vi "move_backlash.vi"(6 "Axis enable":bool[](array[boolean])=[TRUE, TRUE, TRUE, TRUE], 8 "error in":errorcluster, 9 "Axis positions":dbl[](array[numeric]), 10 "Absolute":bool=TRUE, 11 "Trio handle":refnum<k7>) -> (0 "error out":errorcluster, 1 "Final axis errors":i32[](array[numeric]))   [LabVIEW 2024]
panel:
  out "Pull-in errors":dbl[][](graph)
  out "Pull in iterations":i32
  in  "Pull in gain":dbl=0.8
  in  "Clear histogram":bool
  in  "Histogram N":i32=10
  out "Error histogram":cluster{"X":i32[], "Y":i32[]}[](graph)
  in  "Pull in offset":i32=15
  in  "Backlash offset":i32=100
  # "Diagnostics"
  # "The controller axis numbers (starting from 1)"
  # "Like ni_move.vi, but always approaches the position in the + direction.  This minimizes the contribution of backlash to nonrepeatability.  For this to work, pull-in moves must be set to 0 for the axes so that the motion controller won't try to back up."
  # "Parameters:"
  # "Amount we offset position by when approaching from the reverse direction.  Some value greater than the backlash (in steps.)"
  # "Amount we stop short in direction of travel.  Some value (in steps) more than the typical open-loop error, but well less than a full step.  This way our pull-in move is always in the right direction."
  # "Fraction of remaining distance we pull in on each move."
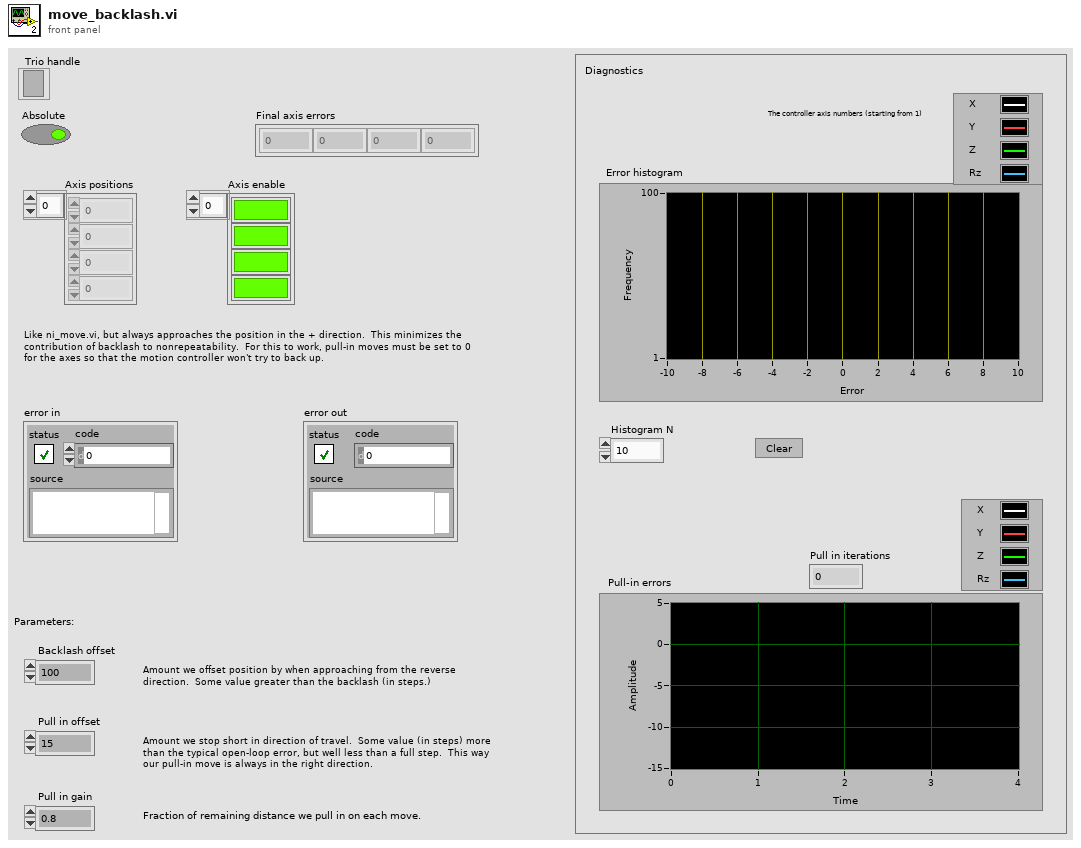
[diagram p1: front panel]
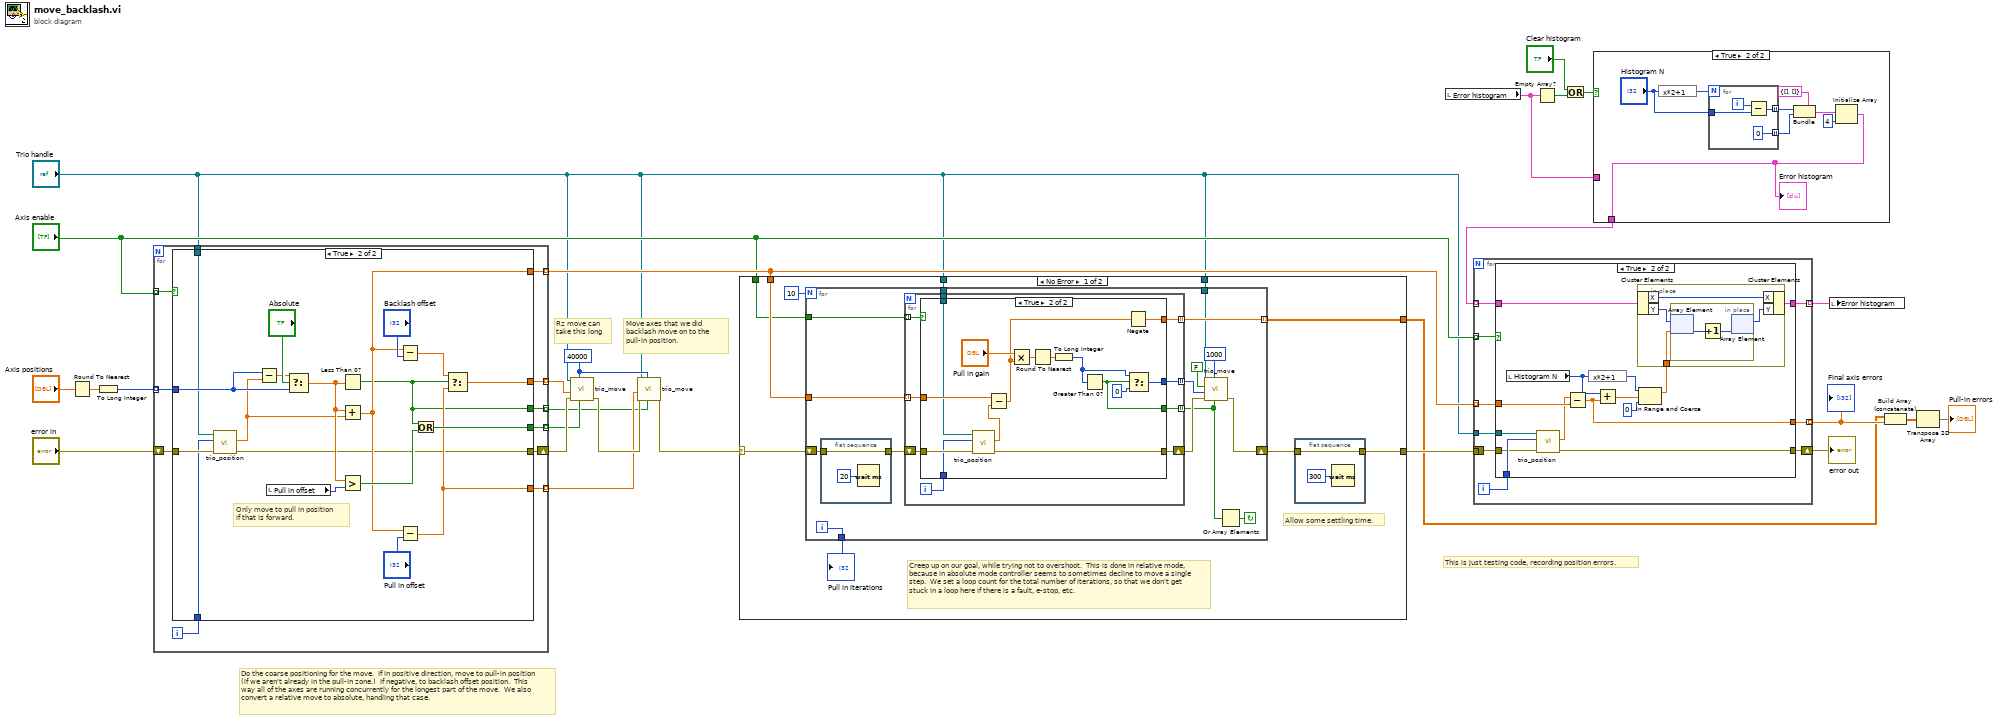
[diagram p0: block diagram]
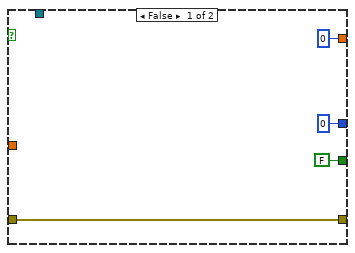
[diagram p2: hidden frame]
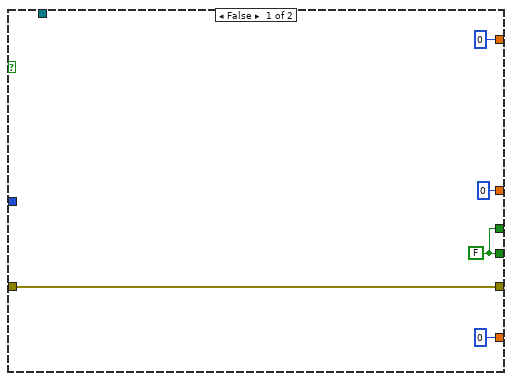
[diagram p4: hidden frame]
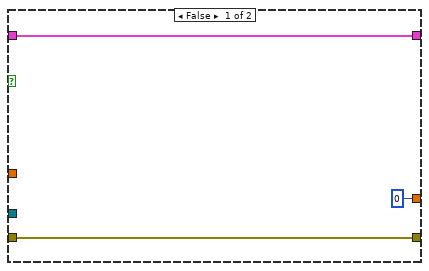
[diagram p6: hidden frame]
diagram:
  w3 = u32 40000 ("Timeout")
  # "Rz move can take this long"
  # "Move axes that we did backlash move on to the pull-in position."
  # "Do the coarse positioning for the move.  If in positive direction, move to pull-in position (if we aren't already in the pull-in zone.)  If negative, to backlash offset position.  This way all of the axes are running concurrently for the longest part of the move.  We also convert a relative move to absolute, handling that case."
  # "This is just testing code, recording position errors."
  n1 = Round To Nearest(number="Axis positions") -> (nearest integer value=w26:dbl[])
  n2 = To Long Integer(number=w26) -> (32bit integer=w24:i32[])
  n3 = for {
    tunnel: "Axis enable" -> [w37] mode=indexing
    tunnel: w24 -> [w36] mode=indexing
    shift-right: [w35] -> w9
    shift-left: "error in" -> [w38]
    tunnel: [w33] -> w7 mode=indexing
    tunnel: [w32] -> w23 mode=indexing
    tunnel: [w31] -> w10 mode=indexing
    tunnel: [w30] -> w6 mode=indexing
    tunnel: [w29] -> w5 mode=indexing
    tunnel: "Trio handle" -> [w28]
    i -> [w34]
    n4 = case shown="True" w37 {
      tunnel: w38 -> [w43 w48]
      tunnel: w34 -> [_ w47]
      tunnel: w36 -> [_ w60]
      tunnel: [w43 w44] -> w35
      tunnel: [w40 w55] -> w33
      tunnel: [0 w53] -> w32
      tunnel: [0 w51] -> w31
      tunnel: [0 w50] -> w30
      tunnel: [w40 w49] -> w29
      tunnel: w28 -> [_ w46]
      frame False {
        w40 = FALSE
      }
      frame True {
        # "Only move to pull in position\nif that is forward."
        n5 = call "trio_position.vi"("error in"=w48, "Axis"=w47, "Trio handle"=w46) -> ("error out"=w44:errorcluster, "Position"=w45:dbl)  [unwired: 6 in, 1 out]
        n6 = Subtract(x=w60, y=w45) -> (x-y=w61:dbl)
        n7 = local read "Pull in offset"() -> (w58:i32)
        n8 = Select(t=w61, s="Absolute", f=w60) -> (s? t:f=w56:dbl)
        n9 = Less Than 0?(x=w56) -> (x < 0?=w49:bool)
        n10 = Add(x=w56, y=w45) -> (x+y=w53:dbl)
        n11 = Greater?(x=w56, y=w58) -> (0:w57:bool)
        n12 = Subtract(x=w53, y="Backlash offset") -> (x-y=w52:dbl)
        n13 = Subtract(x=w53, y="Pull in offset") -> (x-y=w50:dbl)
        n14 = Or(x=w49, y=w57) -> (x .or. y?=w55:bool)
        n15 = Select(t=w52, s=w49, f=w50) -> (s? t:f=w51:dbl)
      }
    }
  }
  n16 = call "trio_move.vi"("Axis enable"=w7, "Timeout (ms)"=w3, "error in"=w9, "Axis positions"=w10, "Trio handle"="Trio handle") -> ("error out"=w8:errorcluster)  [unwired: 5 in, 1 out]
  n17 = call "trio_move.vi"("Axis enable"=w5, "Timeout (ms)"=w3, "error in"=w8, "Axis positions"=w6, "Trio handle"="Trio handle") -> ("error out"=w4:errorcluster)  [unwired: 5 in, 1 out]
  n18 = case shown="No Error" w4 {
    selector: w4 -> [w67 w120]
    tunnel: w23 -> [w72 _]
    tunnel: [w66 w120] -> w20
    tunnel: [w69 _] -> w12
    tunnel: "Axis enable" -> [w68 _]
    tunnel: "Trio handle" -> [w64 _]
    tunnel: "Trio handle" -> [w63 _]
    frame No Error {
      # "Allow some settling time."
      # "Creep up on our goal, while trying not to overshoot.  This is done in relative mode, because in absolute mode controller seems to sometimes decline to move a single step.  We set a loop count for the total number of iterations, so that we don't get stuck in a loop here if there is a fault, e-stop, etc."
      n19 = for {
        N: 10 -> [_]
        tunnel: w68 -> [w87]
        tunnel: w72 -> [w86]
        tunnel: [w83] -> w71
        tunnel: [w78] -> w69 mode=indexing
        shift-right: [w85] -> w65
        shift-left: w67 -> [w80]
        tunnel: w64 -> [w76]
        tunnel: w63 -> [w75]
        i -> [w83]
        stop <- w82 continue-if-true
        n20 = flat-sequence {
          tunnel: w80 -> [w90]
          tunnel: [w90] -> w79
          frame #0 {
            n21 = Wait (ms)(milliseconds to wait=u32 20) -> ()  [unwired: 1 out]
          }
        }
        n22 = for {
          tunnel: w87 -> [w99] mode=indexing
          tunnel: w86 -> [w98] mode=indexing
          shift-right: [w97] -> w89
          shift-left: w79 -> [w100]
          tunnel: [w95] -> w84 mode=indexing
          tunnel: [w94] -> w88 mode=indexing
          tunnel: [w93] -> w78 mode=indexing
          tunnel: w76 -> [w92]
          i -> [w96]
          n23 = case shown="True" w99 {
            tunnel: w100 -> [w104 w109]
            tunnel: w96 -> [_ w108]
            tunnel: w98 -> [_ w116]
            tunnel: [w104 w106] -> w97
            tunnel: [FALSE w119] -> w95
            tunnel: [0 w118] -> w94
            tunnel: [0 w110] -> w93
            tunnel: w92 -> [_ w107]
            frame False {
            }
            frame True {
              n24 = call "trio_position.vi"("error in"=w109, "Axis"=w108, "Trio handle"=w107) -> ("error out"=w106:errorcluster, "Position"=w105:dbl)  [unwired: 6 in, 1 out]
              n25 = Subtract(x=w116, y=w105) -> (x-y=w111:dbl)
              n26 = Multiply(x="Pull in gain", y=w111) -> (x*y=w114:dbl)
              n27 = Round To Nearest(number=w114) -> (nearest integer value=w113:dbl)
              n28 = To Long Integer(number=w113) -> (32bit integer=w112:i32)
              n29 = Greater Than 0?(x=w112) -> (x > 0?=w119:bool)
              n30 = Negate(x=w111) -> (-x=w110:dbl)
              n31 = Select(t=w112, s=w119, f=0) -> (s? t:f=w118:i32)
            }
          }
        }
        n32 = call "trio_move.vi"("Axis enable"=w84, "Timeout (ms)"=u32 1000 ("Timeout"), "error in"=w89, "Axis positions"=w88, "Absolute"=FALSE, "Trio handle"=w75) -> ("error out"=w85:errorcluster)  [unwired: 4 in, 1 out]
        n33 = Or Array Elements(Boolean array=w84) -> (logical OR=w82:bool)
      }
      "Pull in iterations" <- w71
      n34 = flat-sequence {
        tunnel: [w73] -> w66
        tunnel: w65 -> [w73]
        frame #0 {
          n35 = Wait (ms)(milliseconds to wait=u32 300) -> ()  [unwired: 1 out]
        }
      }
    }
    frame Error {
    }
  }
  n36 = local read "Error histogram"() -> (w22:cluster{"X":i32[], "Y":i32[]}[])
  n37 = Empty Array?(array=w22) -> (empty?=w18:bool)
  n38 = Or(x="Clear histogram", y=w18) -> (x .or. y?=w17:bool)
  n39 = case shown="True" w17 {
    tunnel: w22 -> [w121 _]
    tunnel: [w121 w122] -> w21
    frame False {
      # "Histogram initialized"
    }
    frame True {
      n40 = expression code="x*2+1"("Histogram N") -> (w129:i32)
      n41 = for {
        N: w129 -> [_]
        tunnel: "Histogram N" -> [w132]
        tunnel: [w131] -> w127 mode=indexing
        tunnel: [0 ("Histogram N")] -> w126 mode=indexing
        i -> [w133]
        n42 = Subtract(x=w133, y=w132) -> (x-y=w131:i32)
      }
      n43 = Bundle(cluster=cluster{"X":i32[], "Y":i32[]} {"X"=[], "Y"=[]}, "X"=w127, "Y"=w126) -> (w125:cluster{"X":i32[], "Y":i32[]})
      n44 = Initialize Array(w125, 4 ("dimension size")) -> (w122:cluster{"X":i32[], "Y":i32[]}[])
      "Error histogram" <- w122
    }
  }
  n45 = for {
    tunnel: "Axis enable" -> [w142] mode=indexing
    tunnel: w23 -> [w141] mode=indexing
    shift-right: [w135] -> w1
    shift-left: _ -> [w134]
    tunnel: w21 -> [w139] mode=indexing
    tunnel: [w138] -> w16 mode=indexing
    tunnel: w20 -> [_]
    tunnel: [w137] -> w15 mode=indexing
    tunnel: "Trio handle" -> [w136]
    i -> [w140]
    n46 = case shown="True" w142 {
      tunnel: w140 -> [_ w149]
      tunnel: w141 -> [_ w154]
      tunnel: [w143 w148] -> w135
      tunnel: w139 -> [w145 w157]
      tunnel: [w145 w155] -> w138
      tunnel: [0 w153] -> w137
      tunnel: w136 -> [_ w150]
      tunnel: w134 -> [w143 w147]
      frame False {
      }
      frame True {
        n47 = local read "Histogram N"() -> (w152:i32)
        n48 = call "trio_position.vi"("error in"=w147, "Axis"=w149, "Trio handle"=w150) -> ("error out"=w148:errorcluster, "Position"=w146:dbl)  [unwired: 6 in, 1 out]
        n49 = Subtract(x=w146, y=w154) -> (x-y=w153:dbl)
        n50 = expression code="x*2+1"(w152) -> (w151:i32)
        n51 = Add(x=w152, y=w153) -> (x+y=w159:dbl)
        n52 = In Range and Coerce(upper limit=w151, x=w159, lower limit=0) -> (coerced(x)=w156:dbl)  [unwired: 1 out]
        n53 = in-place {
          in-place-border: w156 -> [w161]
          n54 = in-place-cluster #1(w157) -> ("X"=w163:i32[], "Y"=w162:i32[])
          n55 = in-place {
            n56 = in-place-array #2(w162, w161) -> (w165:i32)
            n57 = Increment(x=w165) -> (x+1=w164:i32)
            n58 = in-place-array #2(w164) -> (w160:i32[])  [unwired: 1 out]
          }
          n59 = in-place-cluster #1("X"=w163, "Y"=w160) -> (w155:cluster{"X":i32[], "Y":i32[]})
        }
      }
    }
  }
  "error out" <- w1
  "Final axis errors" <- w15
  n60 = local write "Error histogram"(w16) -> ()
  n61 = Build Array (concatenate)(w12, w15) -> (w14:dbl[][])
  n62 = Transpose 2D Array(2D array=w14) -> (transposed array=→"Pull-in errors":dbl[][])
